vi "Encode_UnsignedThousandths.vi"(1 "Unsigned Thousandths (0.00)":dbl[](array[numeric])) -> (0 "Little Endian":u8[](array[numeric]))   [LabVIEW 2015, in "navX Library v3.lvlib" / "navX Registry Cache.lvclass"]
uses:
  navX Registry Cache.lvclass
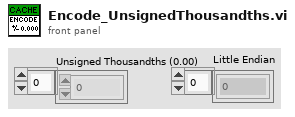
[diagram p1: front panel]
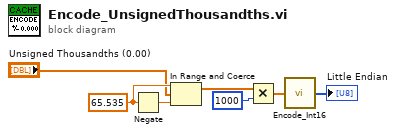
[diagram p0: block diagram]
diagram:
  w6 = 65.535
  n1 = Negate(x=w6) -> (-x=w5:dbl)
  n2 = In Range and Coerce(upper limit=w6, x="Unsigned Thousandths (0.00)", lower limit=w5) -> (coerced(x)=w4:dbl[])  [unwired: 1 out]
  n3 = Multiply(x=w4, y=1000) -> (x*y=w2:dbl[])
  n4 = call "Encode_Int16.vi"("Int16"=w2) -> ("Little Endian"=→"Little Endian":u8[])
